vi "CAN MESSAGE.vi"(3 "data":T1[](array[typedef]) {"payload" format="%x"; "timestamp" format="%<%.7X\n%x>T"; "type" items=["CAN Data"=0, "CAN Remote"=1, "CAN Bus Error"=2, "CAN 2.0 Data"=8, "CAN FD Data"=16, "CAN FD+BRS Data"=24, "J1939 Data"=192, "Delay"=224, "Log Trigger"=225, "Start Trigger"=226]; "identifier" format="%x"}) -> ()   [LabVIEW 2022 SP3]
uses:
  <vilib>/xnet/xnet.llb/XNET Write (Frame CAN).vi
  <vilib>/xnet/xnet.llb/XNET Read (Frame CAN).vi
  <vilib>/xnet/xnet.llb/XNET Create Session (Frame Input Stream).vi
  <vilib>/xnet/xnet.llb/XNET Create Session (Frame Output Queued).vi
  <resource>/objmgr/xnet.rc
  <vilib>/xnet/xnet.llb/XNET Frame Type CAN.ctl
  <vilib>/xnet/xnet.llb/XNET Frame CAN.ctl
panel:
  out "data 2":T1[](array[typedef]) {"payload" format="%x"; "timestamp" format="%<%.7X\n%x>T"; "type" items=["CAN Data"=0, "CAN Remote"=1, "CAN Bus Error"=2, "CAN 2.0 Data"=8, "CAN FD Data"=16, "CAN FD+BRS Data"=24, "J1939 Data"=192, "Delay"=224, "Log Trigger"=225, "Start Trigger"=226]; "identifier" format="%x"}
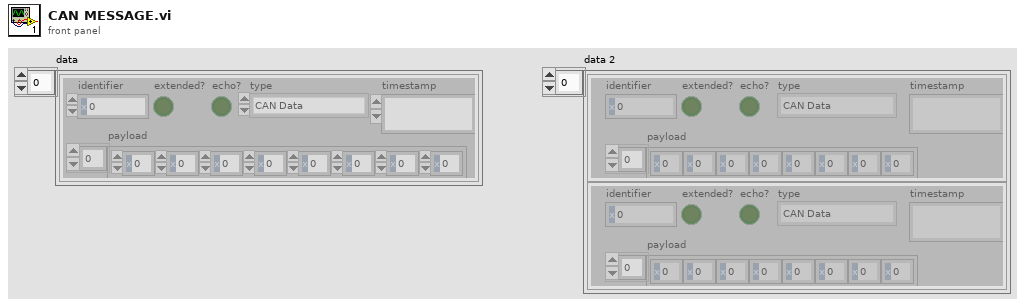
[diagram p1: front panel]
types:
  T1 = typedef "XNET Frame CAN.ctl" = cluster{"timestamp":timestamp, "payload":u8[], "identifier":u32, "type":T2, "extended?":bool, "echo?":bool}
  T2 = typedef "XNET Frame Type CAN.ctl" = u8
  T3 = cluster{"data[0]":T1, "data[1]":T1, "data[2]":T1, "data[3]":T1, "data[4]":T1, "data[5]":T1, "data[6]":T1, "data[7]":T1, "data[8]":T1}
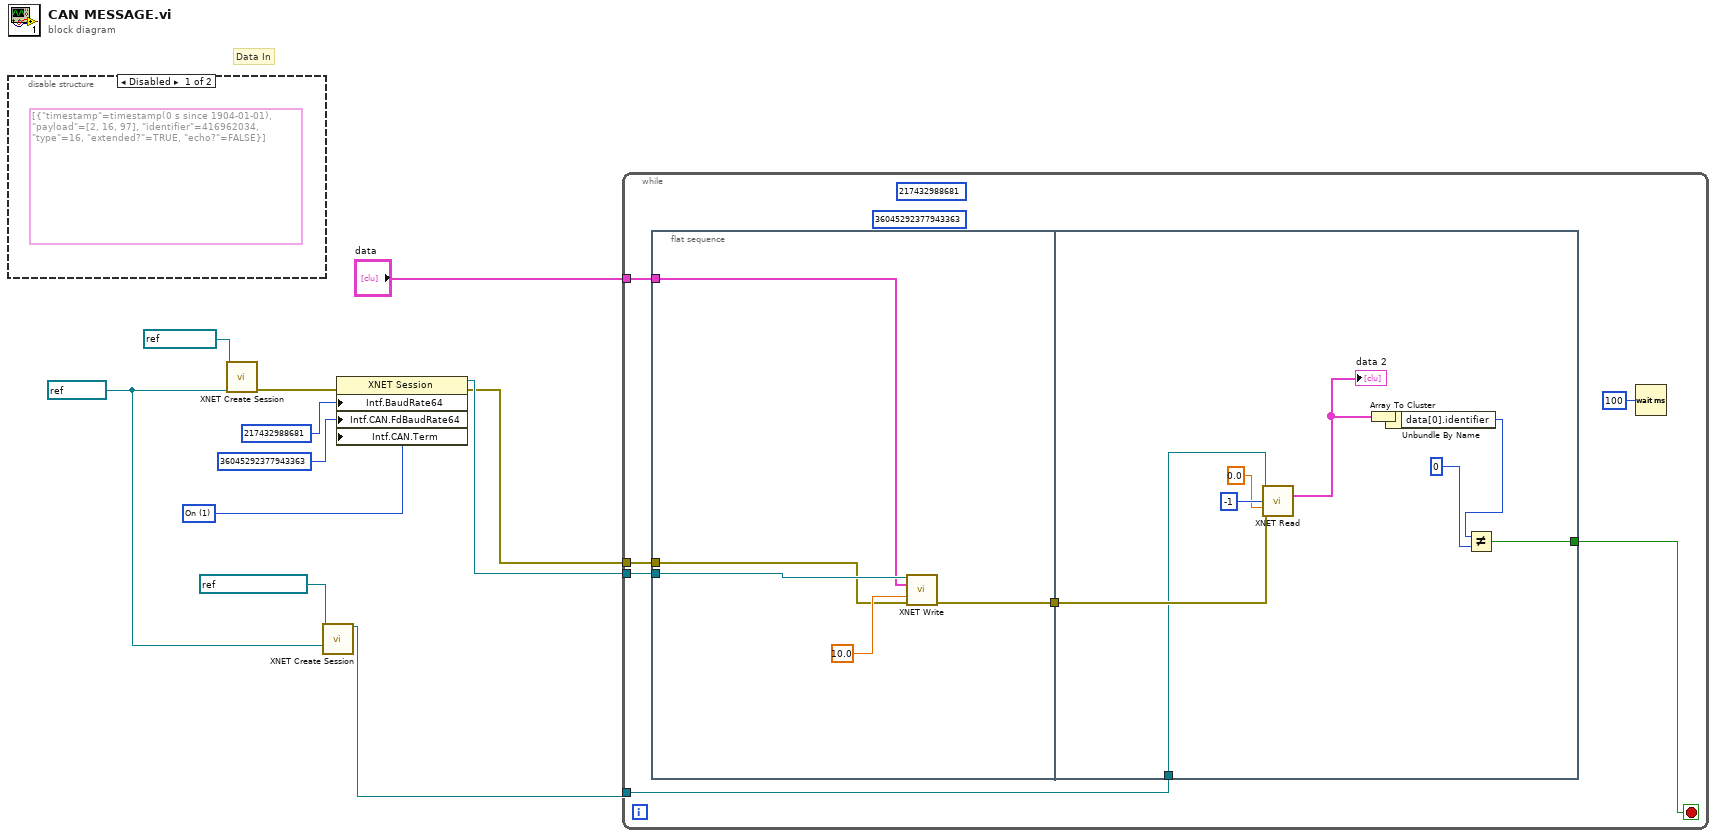
[diagram p0: block diagram]
diagram:
  w2 = u32 1 items=["Off", "On"] ("Interface:CAN:Termination")
  w6 = refnum<k21> "CAN1" ("interface")
  # "Data In"
  n1 = disable-structure shown="Disabled" {
    frame Disabled {
      (unwired) T1[] [{"timestamp"=timestamp(0 s since 1904-01-01), "payload"=[2, 16, 97], "identifier"=416962034, "type"=16, "extended?"=TRUE, "echo?"=FALSE}] ("data")
    }
    frame Enabled {
    }
  }
  n2 = call-poly <vilib>:"XNET Create Session.vi"("frame"=refnum<k21> "Escritura\nElatch_Labview", "interface"=w6) -> ("error out"=w11:errorcluster)  [unwired: 12 in, 1 out]
  n3 = call-poly <vilib>:"XNET Create Session.vi"("cluster (:memory:)"=refnum<k21> "Elatch_Labview", "interface"=w6) -> ("session out"=w8:refnum<k21>)  [unwired: 12 in, 1 out]
  n4 = property class="XNET Session"(error in=w11, "Intf.BaudRate64"=u64 217432988681 ("Interface:64bit Baud Rate"), "Intf.CAN.FdBaudRate64"=u64 36045292377943363 ("Interface:CAN:64bit FD Baud Rate"), "Intf.CAN.Term"=w2) -> (reference out=w4:refnum<k21>, error out=w3:errorcluster)  [unwired: 1 in]
  n5 = while {
    tunnel: w8 -> [w14]
    tunnel: w4 -> [w18]
    tunnel: w3 -> [w17]
    tunnel: "data" -> [w12]
    stop <- w16 stop-if-true
    (unwired) u64 36045292377943363 ("Interface:CAN:64bit FD Baud Rate")
    (unwired) u64 217432988681 ("Interface:64bit Baud Rate")
    n6 = flat-sequence {
      tunnel: w18 -> [w23]
      tunnel: w17 -> [w21]
      tunnel: [w20] -> w15
      tunnel: w12 -> [w19]
      tunnel: [w26] -> w16
      tunnel: w15 -> [w25]
      tunnel: w14 -> [w24]
      frame #0 {
        n7 = call-poly <vilib>:"XNET Write.vi"("session in"=w23, "data"=w19, "timeout (10)"=10.0, "error in (no error)"=w21) -> ("error out"=w20:errorcluster)  [unwired: 10 in, 1 out]
      }
      frame #1 {
        n8 = call-poly <vilib>:"XNET Read.vi"("session in"=w24, "number to read (-1)"=-1, "timeout (0)"=0.0, "error in (no error)"=w25) -> ("data"=w31:T1[])  [unwired: 8 in, 3 out]
        "data 2" <- w31
        n9 = Array To Cluster(array=w31) -> (cluster=w32:T3)
        n10 = Unbundle By Name(w32) -> ("data[0].identifier"=w27:u32)
        n11 = Not Equal?(x=w27, y=u32 0) -> (x != y?=w26:bool)
      }
    }
    n12 = Wait (ms)(milliseconds to wait=u32 100) -> ()  [unwired: 1 out]
  }
